vi "_Copy 1.vi"(0 "XRef":T5, 1 "State In":T1) -> (14 "Reply":T3, 15 "Fatal Error Out":T2, 16 "State Out":T1)   [LabVIEW 2014, in "CSM - Refresh Template.xnode"]
uses:
  CSM - Refresh Template.xnode
  <vilib>/XNodeSupport/XNodeXNodeRef.ctl
  _State 1.ctl
  <vilib>/XNodeSupport/XNodeStringArray.ctl
  <vilib>/XNodeSupport/XNodeString.ctl
  <vilib>/XNodeSupport/XNodeErrorCluster.ctl
  <vilib>/Palette API/Palette Menu/Public Type Define/Palette type.ctl
  <vilib>/XNodeSupport/NI_XNodeSupport.lvlib
  <vilib>/Palette API/Palette Menu/Palette Menu.lvlib
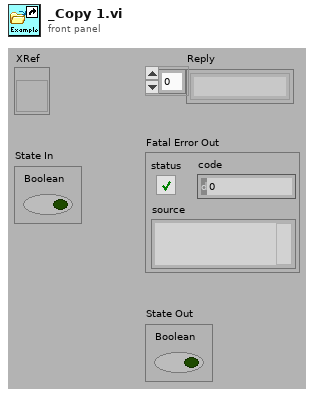
[diagram p1: front panel]
types:
  T1 = typedef "CSM - Refresh Template.xnode/_State 1.ctl" = cluster{"Boolean":bool}
  T2 = typedef "NI_XNodeSupport.lvlib/XNodeErrorCluster.ctl" = errorcluster
  T3 = typedef "NI_XNodeSupport.lvlib/XNodeStringArray.ctl" = T4[]
  T4 = typedef "NI_XNodeSupport.lvlib/XNodeString.ctl" = string
  T5 = typedef "NI_XNodeSupport.lvlib/XNodeXNodeRef.ctl" = refnum<vi>
  T6 = typedef "Palette Menu.lvlib/Palette type.ctl" = i32
  T7 = typedef "Palette Menu.lvlib/Palette Data.ctl" = cluster{"display name":string, "view format":T8, "palette width":i16, "items":T9, "256 color icon":picture, "B&W color icon":picture, "help information":T11, "palette description":string, "synchronize information":T12}
  T8 = typedef "Palette Menu.lvlib/View Format.ctl" = u16
  T9 = typedef "Palette Menu.lvlib/Items.ctl" = T10[]
  T10 = typedef "Palette Menu.lvlib/Item.ctl" = cluster{"item path":path, "library path (.lvlib)":path, "use default lvlib palette":bool, "short name":string, "place VI contents":bool, "hide synchronized item":bool, "reserve spot for synch item":bool, "configure when placing VI contents":bool}
  T11 = typedef "Palette Menu.lvlib/Help Info.ctl" = cluster{"help tag":string, "help file path ":path}
  T12 = typedef "Palette Menu.lvlib/Synchronize Info.ctl" = cluster{"synchronize with directory":bool, "synchronize directory path":path}
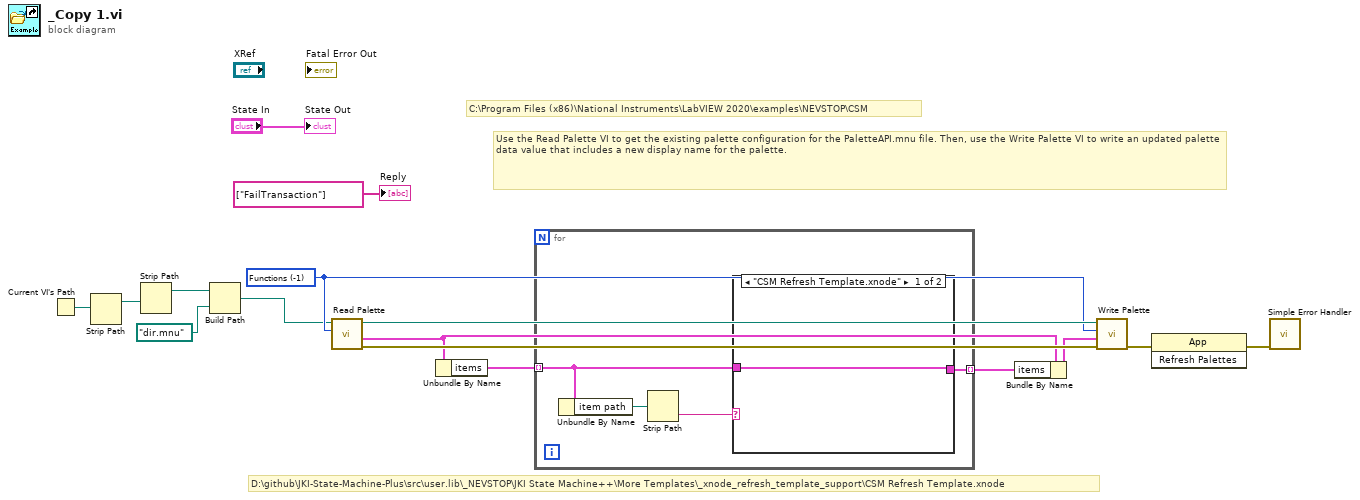
[diagram p0: block diagram]
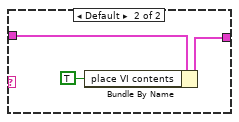
[diagram p2: hidden frame]
diagram:
  w12 = T6 -1 items=["Functions"=-1, "Controls"=-2] ("palette type")
  # "D:\\github\\JKI-State-Machine-Plus\\src\\user.lib\\_NEVSTOP\\JKI State Machine++\\More Templates\\_xnode_refresh_template_support\\CSM Refresh Template.xnode"
  # "Use the Read Palette VI to get the existing palette configuration for the PaletteAPI.mnu file. Then, use the Write Palette VI to write an updated palette data value that includes a new display name for the palette."
  # "C:\\Program Files (x86)\\National Instruments\\LabVIEW 2020\\examples\\NEVSTOP\\CSM"
  n1 = Current VI's Path() -> (path=w9:path)
  n2 = Strip Path(path=w9) -> (stripped path=w8:path)  [unwired: 1 out]
  n3 = Strip Path(path=w8) -> (stripped path=w7:path)  [unwired: 1 out]
  n4 = Build Path(base path=w7, name or relative path=path "dir.mnu") -> (appended path=w11:path)
  n5 = call <vilib>:"Read Palette.vi"("palette type"=w12, "palette path"=w11) -> ("error out"=w14:errorcluster, "palette data"=w6:T7, "duplicate palette path"=w13:path)  [unwired: 2 in, 5 out]
  n6 = Unbundle By Name(w6) -> ("items"=w5:T9)
  n7 = for {
    tunnel: w5 -> [w19] mode=indexing
    tunnel: [w20] -> w4 mode=indexing
    n8 = Unbundle By Name(w19) -> ("item path"=w18:path)
    n9 = Strip Path(path=w18) -> (name=w17:string)  [unwired: 1 out]
    n10 = case shown="\"CSM Refresh Template.xnode\"" w17 {
      tunnel: [w21 w23] -> w20
      tunnel: w19 -> [w21 w22]
      frame "CSM Refresh Template.xnode" {
      }
      frame Default {
        n11 = Bundle By Name(cluster=w22, "place VI contents"=TRUE) -> (w23:T10)
      }
    }
  }
  n12 = Bundle By Name(cluster=w6, "items"=w4) -> (w3:T7)
  n13 = call <vilib>:"Write Palette.vi"("error in (no error)"=w14, "palette data"=w3, "palette type"=w12, "palette path"=w13) -> ("error out"=w1:errorcluster)  [unwired: 1 in, 6 out]
  n14 = invoke class="App" method="Refresh Palettes"(error in=w1) -> (error out=w2:errorcluster)  [unwired: 2 in, 2 out]
  n15 = call <vilib>:"Simple Error Handler.vi"("error in (no error)"=w2) -> ()  [unwired: 1 in, 8 out]
  "Reply" <- T3 ["FailTransaction"] ("Reply")
  "State Out" <- "State In"
